vi "Search Digital Data for Pattern.vi"() -> ()   [LabVIEW 2023]
doc: "Demonstrates the use of the DWDT Search for Digital Pattern VI. A random digital waveform is created and searched for a specified pattern. All pattern matches are displayed in the graph."
uses:
  <vilib>/Waveform/DWDTOps.llb/DWDT Boolean Array to Digital.vi
  <vilib>/Waveform/DWDTOps.llb/DWDT Search for Digital Pattern.vi
panel:
  out "Digital Waveform Graph":digitalwaveform(graph)
  in  "Digital Waveform Pattern":digitalwaveform(waveform)={"t0"=timestamp(0 s since 1904-01-01), "dt"=1.0, "Y"={"transitions"=[], "data"=[[0], [1], [0], [1]]}}
  # "Overview: Searches a random set of digital data for a specified digital pattern.\nInstructions:\nRun the VI. If no instances of the specified pattern are found in the random data, run the VI again."
  # "A random set of digital data is generated and displayed in Digital Waveform Graph. If a sequence of digital values matching Digital Waveform Pattern is found, a cursor will be placed at the start of that sequence of values."
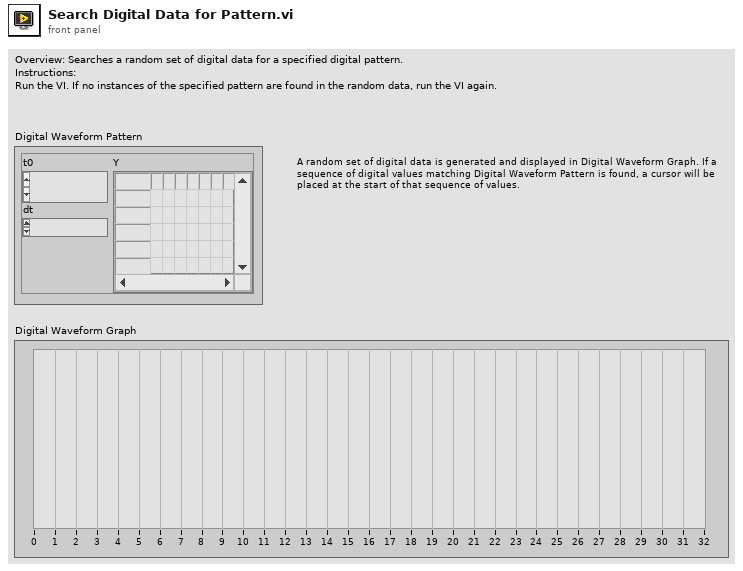
[diagram p1: front panel]
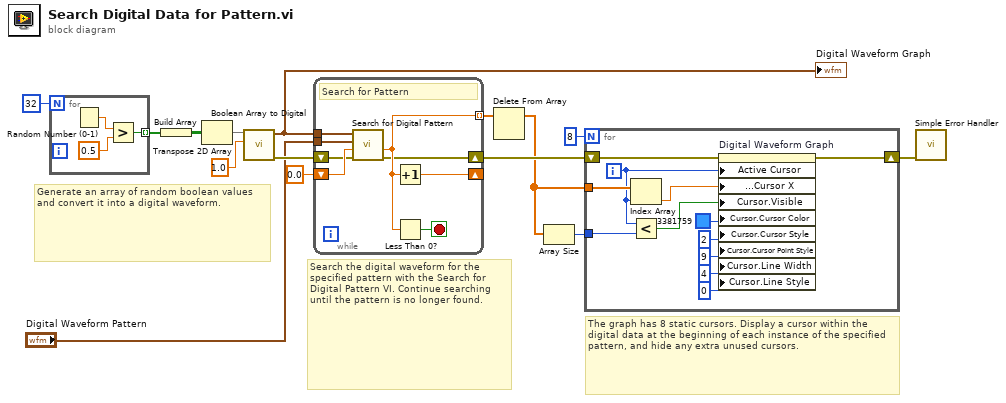
[diagram p0: block diagram]
diagram:
  # "The graph has 8 static cursors. Display a cursor within the digital data at the beginning of each instance of the specified pattern, and hide any extra unused cursors."
  # "Search the digital waveform for the specified pattern with the Search for Digital Pattern VI. Continue searching until the pattern is no longer found."
  # "Generate an array of random boolean values and convert it into a digital waveform."
  n1 = for {
    N: 32 -> [_]
    tunnel: [w16] -> w14 mode=indexing
    n2 = Random Number (0-1)() -> (number: 0 to 1=w18:dbl)
    n3 = Greater?(x=w18, y=0.5) -> (0:w16:bool)
  }
  n4 = Build Array(w14) -> (w13:bool[][])
  n5 = Transpose 2D Array(2D array=w13) -> (transposed array=w4:bool[][])
  n6 = call-poly <vilib>:"Boolean Array to Digital.vi"("sample rate"=1.0, "boolean array"=w4) -> ("error out"=w12:errorcluster, "digital waveform"=w9:digitalwaveform)  [unwired: 8 in]
  "Digital Waveform Graph" <- w9
  n7 = while {
    tunnel: w9 -> [w26]
    tunnel: [w22] -> w8 mode=indexing
    shift-right: [w24] -> _
    shift-left: 0.0 -> [w25]
    shift-right: [w20] -> w7
    shift-left: w12 -> [w21]
    tunnel: "Digital Waveform Pattern" -> [w19]
    stop <- w23 stop-if-true
    # "Search for Pattern"
    n8 = call-poly <vilib>:"Search for Digital Pattern.vi"("error in (no error)"=w21, "start index/time"=w25, "digital pattern"=w19, "digital waveform in"=w26) -> ("error out"=w20:errorcluster, "index/time of pattern"=w22:dbl)  [unwired: 5 in, 1 out]
    n9 = Increment(x=w22) -> (x+1=w24:dbl)
    n10 = Less Than 0?(x=w22) -> (x < 0?=w23:bool)
  }
  n11 = Delete From Array(array=w8) -> (array with subset deleted=w2:dbl[])  [unwired: 2 in, 1 out]
  n12 = Array Size(array=w2) -> (size(s)=w1:i32)
  n13 = for {
    N: 8 -> [_]
    shift-right: [w37] -> w6
    shift-left: w7 -> [w38]
    tunnel: w2 -> [w31]
    tunnel: w1 -> [w28]
    i -> [w29]
    n14 = Index Array(array=w31, index=w29) -> (element=w30:dbl)
    n15 = Less?(x=w29, y=w28) -> (x < y?=w27:bool)
    n16 = property on="Digital Waveform Graph" class="DigitalGraph (strict)"(error in=w38, "Active Cursor"=w29, "Cursor.Cursor Position:Cursor X"=w30, "Cursor.Visible"=w27, "Cursor.Cursor Color"=u32 3381759, "Cursor.Cursor Style"=u8 2, "Cursor.Cursor Point Style"=u8 9, "Cursor.Line Width"=u8 4, "Cursor.Line Style"=u8 0) -> (error out=w37:errorcluster)  [unwired: 1 in, 1 out]
  }
  n17 = call <vilib>:"Simple Error Handler.vi"("error in (no error)"=w6) -> ()  [unwired: 4 in, 5 out]
